vi "Arm - In Position Detector.vi"(8 "error in (no error)":errorcluster, 10 "Current Arm Mode":T1, 11 "AIDeviceRef":T2={"DevStatus"={"status"=FALSE, "code"=0, "source"=""}, "Analog Channel"=enum."Invalid"}) -> (0 "error out":errorcluster, 1 "Current Angle":dbl, 2 "Set Angle":dbl, 3 "Disable Motor":bool, 4 "Set Lock":bool)   [LabVIEW 2015]
uses:
  <vilib>/Rock Robotics/WPI/AnalogChannel/WPI_AnalogChannelDevRef.ctl
  <vilib>/Rock Robotics/SystemInterfaces/AI/FPGA_AIChannel.ctl
  Arm Mode TypeDef.ctl
  Arm Mode LEDs.ctl
  <vilib>/Rock Robotics/Network Tables/NT Read Number.vi
  <vilib>/Rock Robotics/Network Tables/NT Write Number.vi
  Global Variables.vi
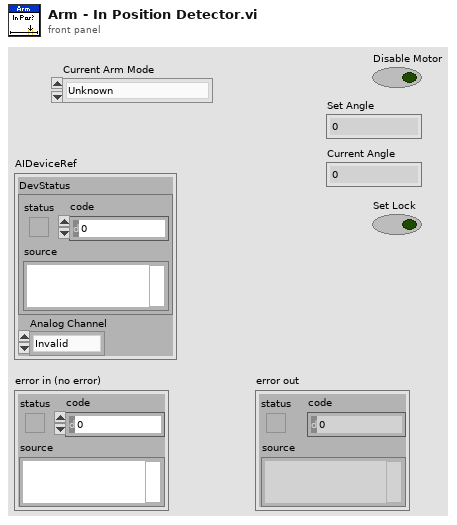
[diagram p1: front panel]
types:
  T1 = typedef "Arm Mode TypeDef.ctl" = enum16{"Unknown", "Disabled", "Locked", "Shoot Batter", "Shoot Close", "Cross Defense", "Human Player Load", "Low Bar / Goal", "Manual"}
  T2 = typedef "WPI_AnalogChannelDevRef.ctl" = cluster{"DevStatus":errorcluster, "Analog Channel":T3}
  T3 = typedef "FPGA_AIChannel.ctl" = enum8{"AI 0", "AI 1", "AI 2", "AI 3", "AI MXP 0", "AI MXP 1", "AI MXP 2", "AI MXP 3", "Invalid"}
  T4 = typedef "Arm Mode LEDs.ctl" = cluster{"Shoot Batter":bool, "Shoot Close":bool, "Shoot Far":bool, "Low Bar / Goal":bool, "Human Player Load":bool, "Manual":bool}
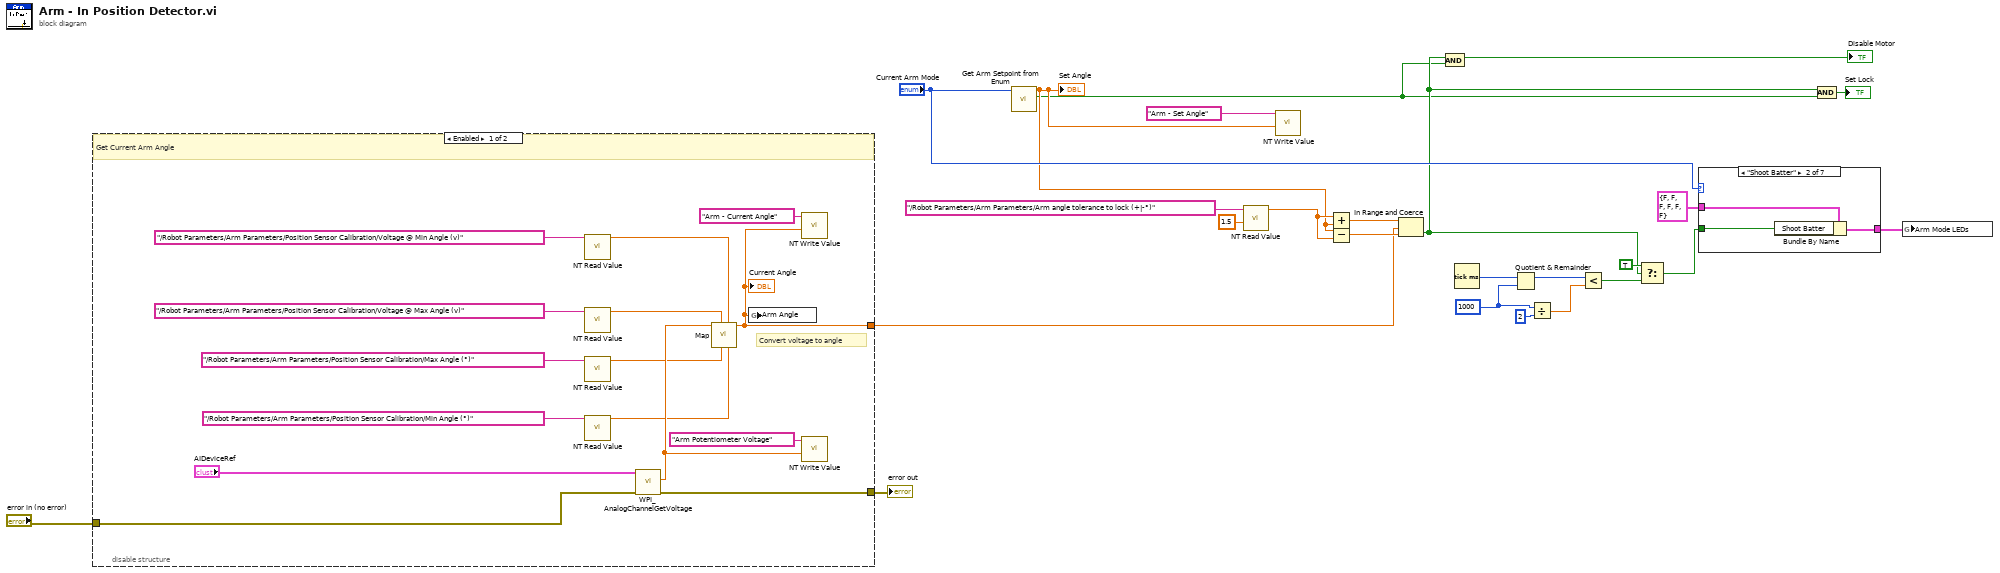
[diagram p0: block diagram]
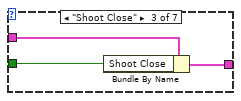
[diagram p4: hidden frame]
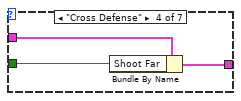
[diagram p5: hidden frame]
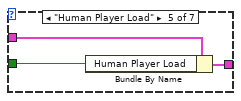
[diagram p6: hidden frame]
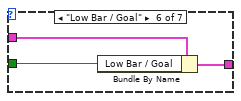
[diagram p7: hidden frame]
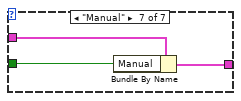
[diagram p8: hidden frame]
diagram:
  w21 = u32 1000 ("y")
  n1 = disable-structure shown="Enabled" {
    disable-tunnel: "error in (no error)" -> [w28 _]
    disable-tunnel: [w27 _] -> w6
    disable-tunnel: [w26 _] -> w5
    frame Enabled {
      # "Convert voltage to angle"
      # "Get Current Arm Angle"
      n2 = call-poly <vilib>:"NT Read Value.vi"("Name"="/Robot Parameters/Arm Parameters/Position Sensor Calibration/Voltage @ Min Angle (v)") -> ("Numeric"=w31:dbl)  [unwired: 9 in, 1 out]
      n3 = call-poly <vilib>:"NT Read Value.vi"("Name"="/Robot Parameters/Arm Parameters/Position Sensor Calibration/Voltage @ Max Angle (v)") -> ("Numeric"=w30:dbl)  [unwired: 9 in, 1 out]
      n4 = call-poly <vilib>:"NT Read Value.vi"("Name"="/Robot Parameters/Arm Parameters/Position Sensor Calibration/Max Angle (°)") -> ("Numeric"=w32:dbl)  [unwired: 9 in, 1 out]
      n5 = call-poly <vilib>:"NT Read Value.vi"("Name"="/Robot Parameters/Arm Parameters/Position Sensor Calibration/Min Angle (°)") -> ("Numeric"=w33:dbl)  [unwired: 9 in, 1 out]
      n6 = call <vilib>:"WPI_AnalogChannelGetVoltage.vi"("error in (no error)"=w28, "AIDeviceRef"="AIDeviceRef") -> ("error out"=w26:errorcluster, "Voltage"=w34:dbl)  [unwired: 7 in, 1 out]
      n7 = call "Map.vi"("Output High"=w33, "Input High"=w31, "Output Low"=w32, "Input Low"=w30, "Input"=w34) -> ("Output"=w27:dbl)  [unwired: 6 in]
      "Current Angle" <- w27
      n8 = global write "Global Variables.vi" "Arm Angle"(w27) -> ()
      n9 = call-poly <vilib>:"NT Write Value.vi"("Numeric"=w27, "Name"="Arm - Current Angle") -> ()  [unwired: 9 in, 1 out]
      n10 = call-poly <vilib>:"NT Write Value.vi"("Numeric"=w34, "Name"="Arm Potentiometer Voltage") -> ()  [unwired: 9 in, 1 out]
    }
    frame Disabled {
    }
  }
  "error out" <- w5
  n11 = call "Get Arm Setpoint from Enum.vi"("Arm Mode"="Current Arm Mode") -> ("Angle"=w7:dbl, "Enable Lock"=w1:bool)  [unwired: 8 in, 1 out]
  "Set Angle" <- w7
  n12 = call-poly <vilib>:"NT Read Value.vi"("Default Value"=1.5, "Name"="/Robot Parameters/Arm Parameters/Arm angle tolerance to lock (+|-°)") -> ("Numeric"=w11:dbl)  [unwired: 8 in, 1 out]
  n13 = call-poly <vilib>:"NT Write Value.vi"("Numeric"=w7, "Name"="Arm - Set Angle") -> ()  [unwired: 9 in, 1 out]
  n14 = Add(x=w11, y=w7) -> (x+y=w18:dbl)
  n15 = Subtract(x=w7, y=w11) -> (x-y=w17:dbl)
  n16 = In Range and Coerce(upper limit=w18, x=w6, lower limit=w17) -> (In Range?=w3:bool)  [unwired: 1 out]
  n17 = And(x=w3, y=w1) -> (x .and. y?=→"Disable Motor":bool)
  n18 = Tick Count (ms)() -> (millisecond timer value=w22:u32)
  n19 = Quotient & Remainder(x=w22, y=w21) -> (x-y*floor(x/y)=w23:u32)  [unwired: 1 out]
  n20 = Divide(x=w21, y=u32 2) -> (x/y=w19:dbl)
  n21 = Less?(x=w23, y=w19) -> (x < y?=w24:bool)
  n22 = Select(t=TRUE, s=w3, f=w24) -> (s? t:f=w13:bool)
  n23 = case shown="\"Shoot Batter\"" "Current Arm Mode" {
    tunnel: T4 {"Shoot Batter"=FALSE, "Shoot Close"=FALSE, "Shoot Far"=FALSE, "Low Bar / Goal"=FALSE, "Human Player Load"=FALSE, "Manual"=FALSE} -> [w41 w44 w47 w50 w53 w56 w59]
    tunnel: [w41 w43 w46 w49 w52 w55 w58] -> w14
    tunnel: w13 -> [_ w42 w45 w48 w51 w54 w57]
    frame Default {
    }
    frame "Shoot Batter" {
      n24 = Bundle By Name(cluster=w44, "Shoot Batter"=w42) -> (w43:T4)
    }
    frame "Shoot Close" {
      n25 = Bundle By Name(cluster=w47, "Shoot Close"=w45) -> (w46:T4)
    }
    frame "Cross Defense" {
      n26 = Bundle By Name(cluster=w50, "Shoot Far"=w48) -> (w49:T4)
    }
    frame "Human Player Load" {
      n27 = Bundle By Name(cluster=w53, "Human Player Load"=w51) -> (w52:T4)
    }
    frame "Low Bar / Goal" {
      n28 = Bundle By Name(cluster=w56, "Low Bar / Goal"=w54) -> (w55:T4)
    }
    frame "Manual" {
      n29 = Bundle By Name(cluster=w59, "Manual"=w57) -> (w58:T4)
    }
  }
  n30 = And(x=w3, y=w1) -> (x .and. y?=→"Set Lock":bool)
  n31 = global write "Global Variables.vi" "Arm Mode LEDs"(w14) -> ()
